vi "FT_EEPROM_Read.vi"(0 "Handle":u32) -> (1 "FT_Status":u32(ring) items=["FT_OK", "FT_INVALID_HANDLE", "FT_DEVICE_NOT_FOUND", "FT_DEVICE_NOT_OPENED", "FT_IO_ERROR", "FT_INSUFFICIENT_RESOURCES", "FT_INVALID_PARAMETER", "FT_INVALID_BAUD_RATE", "FT_DEVICE_NOT_OPENED_FOR_ERASE", "FT_DEVICE_NOT_OPENED_FOR_WRITE", "FT_FAILED_TO_WRITE_DEVICE", "FT_EEPROM_READ_FAILED", "FT_EEPROM_WRITE_FAILED", "FT_EEPROM_ERASE_FAILED", "FT_EEPROM_NOT_PRESENT", "FT_EEPROM_NOT_PROGRAMMED", "FT_INVALID_ARGS", "FT_NOT_SUPPORTED", "FT_OTHER_ERROR"], 2 "FT232-FT245 EEPROM Contents 4":T2, 3 "output cluster":T1)   [LabVIEW 2019, in "D2XX_HeaterStage.lvlib"]
uses:
  D2XX_HeaterStage.lvlib
  <userlib>/LevyLab/Relay Box/D2XX_Functions/i386/ftd2xx.dll
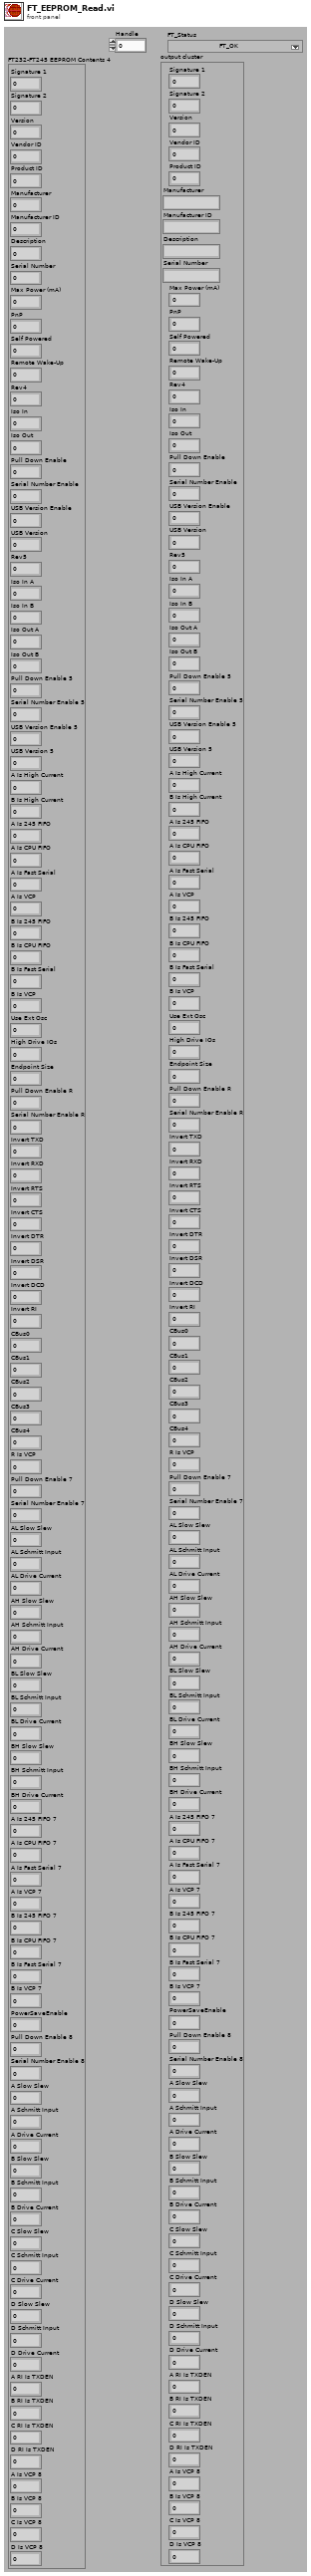
[diagram p1: front panel]
types:
  T1 = cluster{"Signature 1":u32, "Signature 2":u32, "Version":u32, "Vendor ID":u16, "Product ID":u16, "Manufacturer":string, "Manufacturer ID":string, "Description":string, "Serial Number":string, "Max Power (mA)":u16, "PnP":u16, "Self Powered":u16, "Remote Wake-Up":u16, "Rev4":u8, "Iso In":u8, "Iso Out":u8, "Pull Down Enable":u8, "Serial Number Enable":u8, "USB Version Enable":u8, "USB Version":u16, "Rev5":u8, "Iso In A":u8, "Iso In B":u8, "Iso Out A":u8, "Iso Out B":u8, "Pull Down Enable 5":u8, "Serial Number Enable 5":u8, "USB Version Enable 5":u8, "USB Version 5":u16, "A Is High Current":u8, "B Is High Current":u8, "A Is 245 FIFO":u8, "A Is CPU FIFO":u8, "A Is Fast Serial":u8, "A Is VCP":u8, "B Is 245 FIFO":u8, "B Is CPU FIFO":u8, "B Is Fast Serial":u8, "B Is VCP":u8, "Use Ext Osc":u8, "High Drive IOs":u8, "Endpoint Size":u8, "Pull Down Enable R":u8, "Serial Number Enable R":u8, "Invert TXD":u8, "Invert RXD":u8, "Invert RTS":u8, "Invert CTS":u8, "Invert DTR":u8, "Invert DSR":u8, "Invert DCD":u8, "Invert RI":u8, "CBus0":u8, "CBus1":u8, "CBus2":u8, "CBus3":u8, "CBus4":u8, "R Is VCP":u8, "Pull Down Enable 7":u8, "Serial Number Enable 7":u8, "AL Slow Slew":u8, "AL Schmitt Input":u8, "AL Drive Current":u8, "AH Slow Slew":u8, "AH Schmitt Input":u8, "AH Drive Current":u8, "BL Slow Slew":u8, "BL Schmitt Input":u8, "BL Drive Current":u8, "BH Slow Slew":u8, "BH Schmitt Input":u8, "BH Drive Current":u8, "A Is 245 FIFO 7":u8, "A Is CPU FIFO 7":u8, "A Is Fast Serial 7":u8, "A Is VCP 7":u8, "B Is 245 FIFO 7":u8, "B Is CPU FIFO 7":u8, "B Is Fast Serial 7":u8, "B Is VCP 7":u8, "PowerSaveEnable":u8, "Pull Down Enable 8":u8, "Serial Number Enable 8":u8, "A Slow Slew":u8, "A Schmitt Input":u8, "A Drive Current":u8, "B Slow Slew":u8, "B Schmitt Input":u8, "B Drive Current":u8, "C Slow Slew":u8, "C Schmitt Input":u8, "C Drive Current":u8, "D Slow Slew":u8, "D Schmitt Input":u8, "D Drive Current":u8, "A RI Is TXDEN":u8, "B RI Is TXDEN":u8, "C RI Is TXDEN":u8, "D RI Is TXDEN":u8, "A Is VCP 8":u8, "B Is VCP 8":u8, "C Is VCP 8":u8, "D Is VCP 8":u8}
  T2 = cluster{"Signature 1":u32, "Signature 2":u32, "Version":u32, "Vendor ID":u16, "Product ID":u16, "Manufacturer":u32, "Manufacturer ID":u32, "Description":u32, "Serial Number":u32, "Max Power (mA)":u16, "PnP":u16, "Self Powered":u16, "Remote Wake-Up":u16, "Rev4":u8, "Iso In":u8, "Iso Out":u8, "Pull Down Enable":u8, "Serial Number Enable":u8, "USB Version Enable":u8, "USB Version":u16, "Rev5":u8, "Iso In A":u8, "Iso In B":u8, "Iso Out A":u8, "Iso Out B":u8, "Pull Down Enable 5":u8, "Serial Number Enable 5":u8, "USB Version Enable 5":u8, "USB Version 5":u16, "A Is High Current":u8, "B Is High Current":u8, "A Is 245 FIFO":u8, "A Is CPU FIFO":u8, "A Is Fast Serial":u8, "A Is VCP":u8, "B Is 245 FIFO":u8, "B Is CPU FIFO":u8, "B Is Fast Serial":u8, "B Is VCP":u8, "Use Ext Osc":u8, "High Drive IOs":u8, "Endpoint Size":u8, "Pull Down Enable R":u8, "Serial Number Enable R":u8, "Invert TXD":u8, "Invert RXD":u8, "Invert RTS":u8, "Invert CTS":u8, "Invert DTR":u8, "Invert DSR":u8, "Invert DCD":u8, "Invert RI":u8, "CBus0":u8, "CBus1":u8, "CBus2":u8, "CBus3":u8, "CBus4":u8, "R Is VCP":u8, "Pull Down Enable 7":u8, "Serial Number Enable 7":u8, "AL Slow Slew":u8, "AL Schmitt Input":u8, "AL Drive Current":u8, "AH Slow Slew":u8, "AH Schmitt Input":u8, "AH Drive Current":u8, "BL Slow Slew":u8, "BL Schmitt Input":u8, "BL Drive Current":u8, "BH Slow Slew":u8, "BH Schmitt Input":u8, "BH Drive Current":u8, "A Is 245 FIFO 7":u8, "A Is CPU FIFO 7":u8, "A Is Fast Serial 7":u8, "A Is VCP 7":u8, "B Is 245 FIFO 7":u8, "B Is CPU FIFO 7":u8, "B Is Fast Serial 7":u8, "B Is VCP 7":u8, "PowerSaveEnable":u8, "Pull Down Enable 8":u8, "Serial Number Enable 8":u8, "A Slow Slew":u8, "A Schmitt Input":u8, "A Drive Current":u8, "B Slow Slew":u8, "B Schmitt Input":u8, "B Drive Current":u8, "C Slow Slew":u8, "C Schmitt Input":u8, "C Drive Current":u8, "D Slow Slew":u8, "D Schmitt Input":u8, "D Drive Current":u8, "A RI Is TXDEN":u8, "B RI Is TXDEN":u8, "C RI Is TXDEN":u8, "D RI Is TXDEN":u8, "A Is VCP 8":u8, "B Is VCP 8":u8, "C Is VCP 8":u8, "D Is VCP 8":u8}
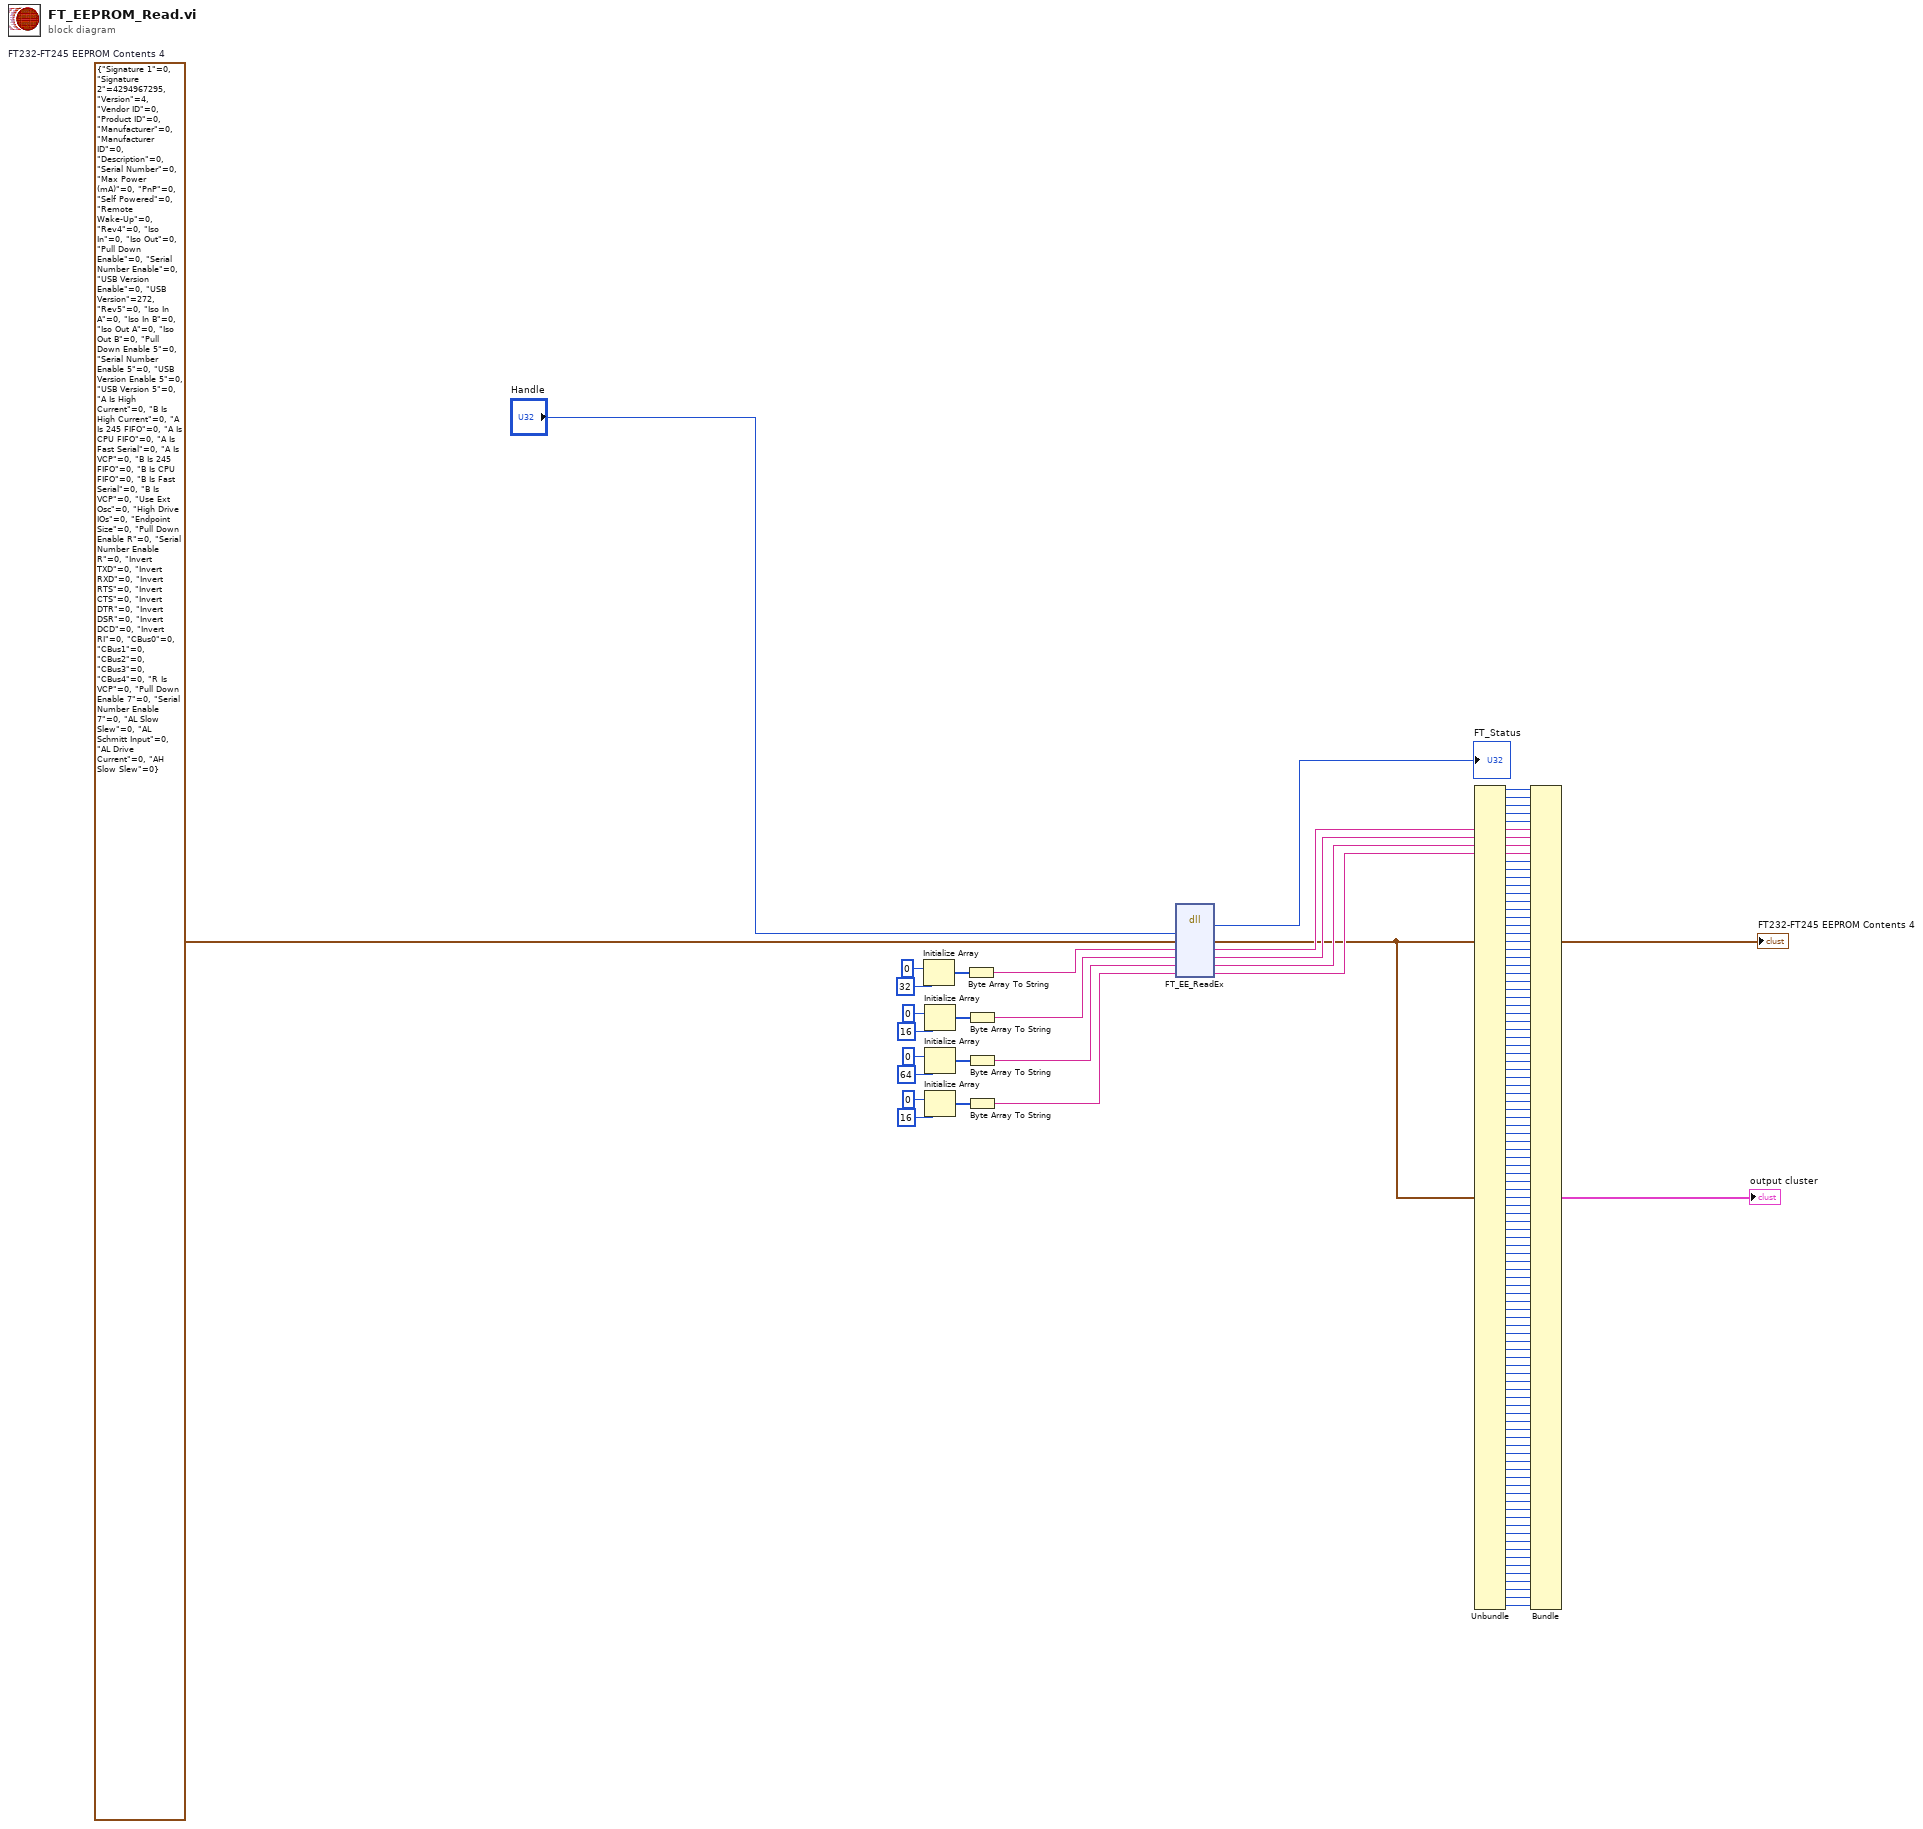
[diagram p0: block diagram]
diagram:
  w100 = T2 {"Signature 1"=0, "Signature 2"=4294967295, "Version"=4, "Vendor ID"=0, "Product ID"=0, "Manufacturer"=0, "Manufacturer ID"=0, "Description"=0, "Serial Number"=0, "Max Power (mA)"=0, "PnP"=0, "Self Powered"=0, "Remote Wake-Up"=0, "Rev4"=0, "Iso In"=0, "Iso Out"=0, "Pull Down Enable"=0, "Serial Number Enable"=0, "USB Version Enable"=0, "USB Version"=272, "Rev5"=0, "Iso In A"=0, "Iso In B"=0, "Iso Out A"=0, "Iso Out B"=0, "Pull Down Enable 5"=0, "Serial Number Enable 5"=0, "USB Version Enable 5"=0, "USB Version 5"=0, "A Is High Current"=0, "B Is High Current"=0, "A Is 245 FIFO"=0, "A Is CPU FIFO"=0, "A Is Fast Serial"=0, "A Is VCP"=0, "B Is 245 FIFO"=0, "B Is CPU FIFO"=0, "B Is Fast Serial"=0, "B Is VCP"=0, "Use Ext Osc"=0, "High Drive IOs"=0, "Endpoint Size"=0, "Pull Down Enable R"=0, "Serial Number Enable R"=0, "Invert TXD"=0, "Invert RXD"=0, "Invert RTS"=0, "Invert CTS"=0, "Invert DTR"=0, "Invert DSR"=0, "Invert DCD"=0, "Invert RI"=0, "CBus0"=0, "CBus1"=0, "CBus2"=0, "CBus3"=0, "CBus4"=0, "R Is VCP"=0, "Pull Down Enable 7"=0, "Serial Number Enable 7"=0, "AL Slow Slew"=0, "AL Schmitt Input"=0, "AL Drive Current"=0, "AH Slow Slew"=0, "AH Schmitt Input"=0, "AH Drive Current"=0, "BL Slow Slew"=0, "BL Schmitt Input"=0, "BL Drive Current"=0, "BH Slow Slew"=0, "BH Schmitt Input"=0, "BH Drive Current"=0, "A Is 245 FIFO 7"=0, "A Is CPU FIFO 7"=0, "A Is Fast Serial 7"=0, "A Is VCP 7"=0, "B Is 245 FIFO 7"=0, "B Is CPU FIFO 7"=0, "B Is Fast Serial 7"=0, "B Is VCP 7"=0, "PowerSaveEnable"=0, "Pull Down Enable 8"=0, "Serial Number Enable 8"=0, "A Slow Slew"=0, "A Schmitt Input"=0, "A Drive Current"=0, "B Slow Slew"=0, "B Schmitt Input"=0, "B Drive Current"=0, "C Slow Slew"=0, "C Schmitt Input"=0, "C Drive Current"=0, "D Slow Slew"=0, "D Schmitt Input"=0, "D Drive Current"=0, "A RI Is TXDEN"=0, "B RI Is TXDEN"=0, "C RI Is TXDEN"=0, "D RI Is TXDEN"=0, "A Is VCP 8"=0, "B Is VCP 8"=0, "C Is VCP 8"=0, "D Is VCP 8"=0}  # FT232-FT245 EEPROM Contents 4
  n1 = Initialize Array(u8 0, 32 ("dimension size")) -> (w121:u8[])
  n2 = Initialize Array(u8 0, 16 ("dimension size")) -> (w119:u8[])
  n3 = Initialize Array(u8 0, 64 ("dimension size")) -> (w117:u8[])
  n4 = Initialize Array(u8 0, 16 ("dimension size")) -> (w115:u8[])
  n5 = Byte Array To String(unsigned byte array=w121) -> (string=w110:string)
  n6 = Byte Array To String(unsigned byte array=w119) -> (string=w109:string)
  n7 = Byte Array To String(unsigned byte array=w117) -> (string=w108:string)
  n8 = Byte Array To String(unsigned byte array=w115) -> (string=w107:string)
  n9 = dll-call lib="C:/Program Files (x86)/National Instruments/LabVIEW 2019/user.lib/LevyLab/Relay Box/D2XX_Functions/i386/FTD2XX.dll" fn="FT_EE_ReadEx"("Handle"="Handle", "FT232-FT245 EEPROM Contents 4"=w100, "Manufacturer"=w110, "Manufacturer ID"=w109, "Description"=w108, "Serial Number"=w107) -> ("FT_Status"=→"FT_Status":u32, "FT232-FT245 EEPROM Contents 4"=w1:T2, "Manufacturer"=w5:string, "Manufacturer ID"=w4:string, "Description"=w3:string, "Serial Number"=w2:string)  [unwired: 4 in, 2 out]
  "FT232-FT245 EEPROM Contents 4" <- w1
  n10 = Unbundle(w1) -> ("Signature 1"=w99:u32, "Signature 2"=w98:u32, "Version"=w97:u32, "Vendor ID"=w106:u16, "Product ID"=w105:u16, "Max Power (mA)"=w104:u16, "PnP"=w103:u16, "Self Powered"=w102:u16, "Remote Wake-Up"=w101:u16, "Rev4"=w96:u8, "Iso In"=w95:u8, "Iso Out"=w94:u8, "Pull Down Enable"=w93:u8, "Serial Number Enable"=w92:u8, "USB Version Enable"=w91:u8, "USB Version"=w90:u16, "Rev5"=w89:u8, "Iso In A"=w88:u8, "Iso In B"=w87:u8, "Iso Out A"=w86:u8, "Iso Out B"=w85:u8, "Pull Down Enable 5"=w84:u8, "Serial Number Enable 5"=w83:u8, "USB Version Enable 5"=w82:u8, "USB Version 5"=w81:u16, "A Is High Current"=w80:u8, "B Is High Current"=w79:u8, "A Is 245 FIFO"=w78:u8, "A Is CPU FIFO"=w77:u8, "A Is Fast Serial"=w76:u8, "A Is VCP"=w75:u8, "B Is 245 FIFO"=w74:u8, "B Is CPU FIFO"=w73:u8, "B Is Fast Serial"=w72:u8, "B Is VCP"=w71:u8, "Use Ext Osc"=w70:u8, "High Drive IOs"=w69:u8, "Endpoint Size"=w68:u8, "Pull Down Enable R"=w67:u8, "Serial Number Enable R"=w66:u8, "Invert TXD"=w65:u8, "Invert RXD"=w64:u8, "Invert RTS"=w63:u8, "Invert CTS"=w62:u8, "Invert DTR"=w61:u8, "Invert DSR"=w60:u8, "Invert DCD"=w59:u8, "Invert RI"=w58:u8, "CBus0"=w57:u8, "CBus1"=w56:u8, "CBus2"=w55:u8, "CBus3"=w54:u8, "CBus4"=w53:u8, "R Is VCP"=w52:u8, "Pull Down Enable 7"=w51:u8, "Serial Number Enable 7"=w50:u8, "AL Slow Slew"=w49:u8, "AL Schmitt Input"=w48:u8, "AL Drive Current"=w47:u8, "AH Slow Slew"=w46:u8, "AH Schmitt Input"=w45:u8, "AH Drive Current"=w44:u8, "BL Slow Slew"=w43:u8, "BL Schmitt Input"=w42:u8, "BL Drive Current"=w41:u8, "BH Slow Slew"=w39:u8, "BH Schmitt Input"=w40:u8, "BH Drive Current"=w38:u8, "A Is 245 FIFO 7"=w37:u8, "A Is CPU FIFO 7"=w36:u8, "A Is Fast Serial 7"=w35:u8, "A Is VCP 7"=w34:u8, "B Is 245 FIFO 7"=w33:u8, "B Is CPU FIFO 7"=w31:u8, "B Is Fast Serial 7"=w32:u8, "B Is VCP 7"=w30:u8, "PowerSaveEnable"=w29:u8, "Pull Down Enable 8"=w28:u8, "Serial Number Enable 8"=w27:u8, "A Slow Slew"=w26:u8, "A Schmitt Input"=w24:u8, "A Drive Current"=w25:u8, "B Slow Slew"=w23:u8, "B Schmitt Input"=w22:u8, "B Drive Current"=w21:u8, "C Slow Slew"=w20:u8, "C Schmitt Input"=w19:u8, "C Drive Current"=w18:u8, "D Slow Slew"=w17:u8, "D Schmitt Input"=w16:u8, "D Drive Current"=w15:u8, "A RI Is TXDEN"=w14:u8, "B RI Is TXDEN"=w13:u8, "C RI Is TXDEN"=w12:u8, "D RI Is TXDEN"=w11:u8, "A Is VCP 8"=w10:u8, "B Is VCP 8"=w8:u8, "C Is VCP 8"=w9:u8, "D Is VCP 8"=w7:u8)  [unwired: 4 out]
  n11 = Bundle("Signature 1"=w99, "Signature 2"=w98, "Version"=w97, "Vendor ID"=w106, "Product ID"=w105, "Manufacturer"=w5, "Manufacturer ID"=w4, "Description"=w3, "Serial Number"=w2, "Max Power (mA)"=w104, "PnP"=w103, "Self Powered"=w102, "Remote Wake-Up"=w101, "Rev4"=w96, "Iso In"=w95, "Iso Out"=w94, "Pull Down Enable"=w93, "Serial Number Enable"=w92, "USB Version Enable"=w91, "USB Version"=w90, "Rev5"=w89, "Iso In A"=w88, "Iso In B"=w87, "Iso Out A"=w86, "Iso Out B"=w85, "Pull Down Enable 5"=w84, "Serial Number Enable 5"=w83, "USB Version Enable 5"=w82, "USB Version 5"=w81, "A Is High Current"=w80, "B Is High Current"=w79, "A Is 245 FIFO"=w78, "A Is CPU FIFO"=w77, "A Is Fast Serial"=w76, "A Is VCP"=w75, "B Is 245 FIFO"=w74, "B Is CPU FIFO"=w73, "B Is Fast Serial"=w72, "B Is VCP"=w71, "Use Ext Osc"=w70, "High Drive IOs"=w69, "Endpoint Size"=w68, "Pull Down Enable R"=w67, "Serial Number Enable R"=w66, "Invert TXD"=w65, "Invert RXD"=w64, "Invert RTS"=w63, "Invert CTS"=w62, "Invert DTR"=w61, "Invert DSR"=w60, "Invert DCD"=w59, "Invert RI"=w58, "CBus0"=w57, "CBus1"=w56, "CBus2"=w55, "CBus3"=w54, "CBus4"=w53, "R Is VCP"=w52, "Pull Down Enable 7"=w51, "Serial Number Enable 7"=w50, "AL Slow Slew"=w49, "AL Schmitt Input"=w48, "AL Drive Current"=w47, "AH Slow Slew"=w46, "AH Schmitt Input"=w45, "AH Drive Current"=w44, "BL Slow Slew"=w43, "BL Schmitt Input"=w42, "BL Drive Current"=w41, "BH Slow Slew"=w39, "BH Schmitt Input"=w40, "BH Drive Current"=w38, "A Is 245 FIFO 7"=w37, "A Is CPU FIFO 7"=w36, "A Is Fast Serial 7"=w35, "A Is VCP 7"=w34, "B Is 245 FIFO 7"=w33, "B Is CPU FIFO 7"=w31, "B Is Fast Serial 7"=w32, "B Is VCP 7"=w30, "PowerSaveEnable"=w29, "Pull Down Enable 8"=w28, "Serial Number Enable 8"=w27, "A Slow Slew"=w26, "A Schmitt Input"=w24, "A Drive Current"=w25, "B Slow Slew"=w23, "B Schmitt Input"=w22, "B Drive Current"=w21, "C Slow Slew"=w20, "C Schmitt Input"=w19, "C Drive Current"=w18, "D Slow Slew"=w17, "D Schmitt Input"=w16, "D Drive Current"=w15, "A RI Is TXDEN"=w14, "B RI Is TXDEN"=w13, "C RI Is TXDEN"=w12, "D RI Is TXDEN"=w11, "A Is VCP 8"=w10, "B Is VCP 8"=w8, "C Is VCP 8"=w9, "D Is VCP 8"=w7) -> (→"output cluster":T1)  [unwired: 1 in]
